vi "Optionen Cluster Anordnen.vi"(8 "error in (no error)":errorcluster caption="Fehler (Eingang, kein Fehler)", 11 "Cluster (Eingang)":refnum<vi>) -> (0 "error out":errorcluster caption="Fehler (Ausgang)", 3 "Numerisch":i32)   [LabVIEW 2020, in "System Einstellungen V2.lvlib"]
uses:
  System Einstellungen V2.lvlib
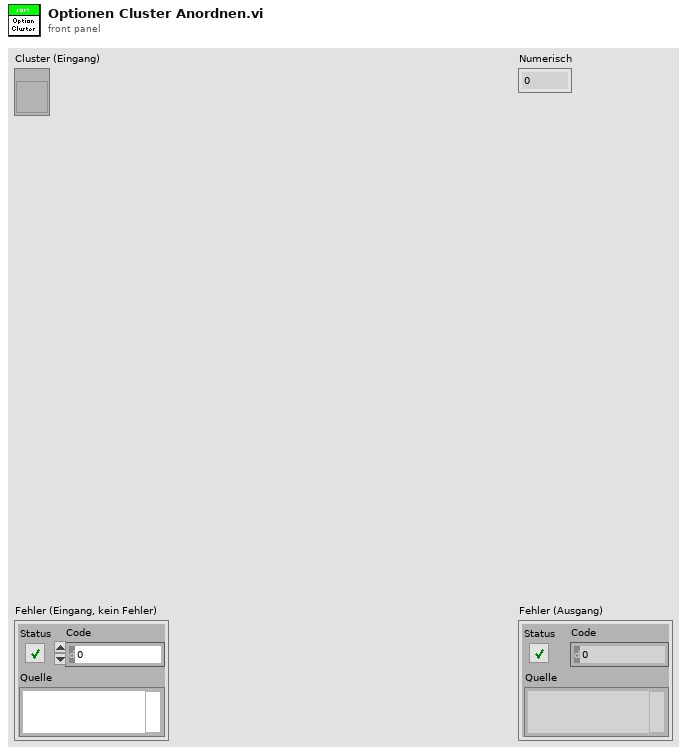
[diagram p1: front panel]
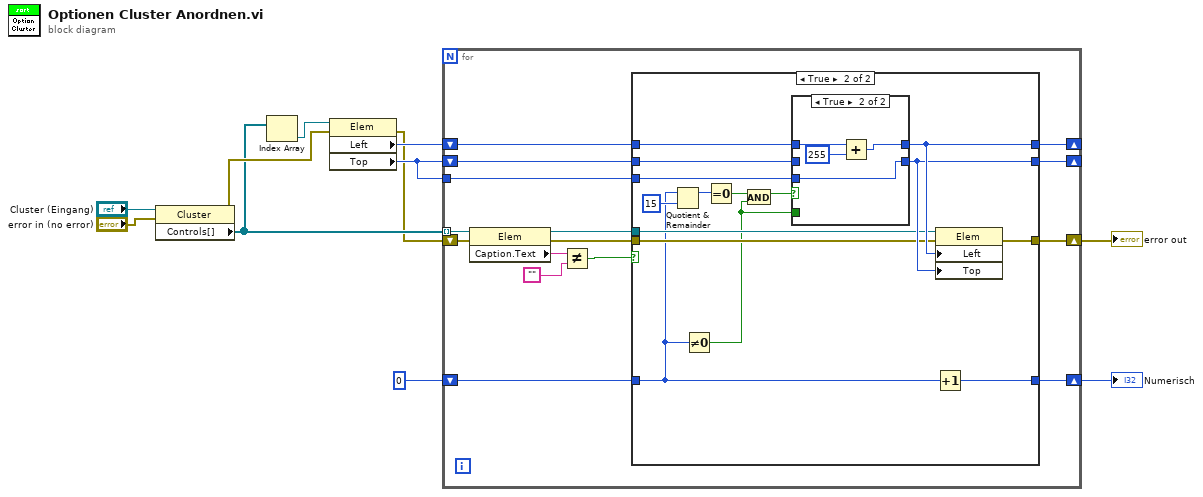
[diagram p0: block diagram]
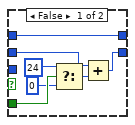
[diagram p3: hidden frame]
diagram:
  n1 = property class="Cluster"(reference="Cluster (Eingang)", error in="error in (no error)") -> (error out=w9:errorcluster, "Controls[]"=w7:refnum<vi>[])  [unwired: 1 out]
  n2 = Index Array(array=w7) -> (element=w10:refnum<vi>)  [unwired: 1 in]
  n3 = property class="Elem"(reference=w10, error in=w9) -> (error out=w3:errorcluster, "Left"=w6:i32, "Top"=w4:i32)  [unwired: 1 out]
  n4 = for {
    tunnel: w7 -> [w18] mode=indexing
    shift-right: [w26] -> w5
    shift-left: w3 -> [w17]
    shift-right: [w23] -> _
    shift-left: w6 -> [w25]
    shift-right: [w22] -> _
    shift-left: w4 -> [w24]
    tunnel: w4 -> [w21]
    shift-right: [w14] -> w1
    shift-left: 0 -> [w16]
    n5 = property class="Elem"(reference=w18, error in=w17) -> (reference out=w12:refnum<vi>, error out=w13:errorcluster, "Caption.Text"=w20:string)
    n6 = Not Equal?(x=w20, y="") -> (x != y?=w15:bool)
    n7 = case shown="True" w15 {
      tunnel: [w29 w45] -> w26
      tunnel: w25 -> [w28 w41]
      tunnel: w24 -> [w27 w40]
      tunnel: [w28 w39] -> w23
      tunnel: [w27 w38] -> w22
      tunnel: w21 -> [_ w37]
      tunnel: w16 -> [w30 w33]
      tunnel: [w30 w36] -> w14
      tunnel: w13 -> [w29 w35]
      tunnel: w12 -> [_ w34]
      frame False {
      }
      frame True {
        n8 = Quotient & Remainder(x=w33, y=15) -> (x-y*floor(x/y)=w43:i32)  [unwired: 1 out]
        n9 = Not Equal To 0?(x=w33) -> (x != 0?=w31:bool)
        n10 = Equal To 0?(x=w43) -> (x = 0?=w42:bool)
        n11 = And(x=w42, y=w31) -> (x .and. y?=w32:bool)
        n12 = case shown="True" w32 {
          tunnel: w41 -> [w52 w55]
          tunnel: w40 -> [w51 _]
          tunnel: [w52 w53] -> w39
          tunnel: [w50 w56] -> w38
          tunnel: w37 -> [_ w56]
          tunnel: w31 -> [w48 _]
          frame False {
            n13 = Select(t=24 ("y"), s=w48, f=0) -> (s? t:f=w49:i32)
            n14 = Add(x=w51, y=w49) -> (x+y=w50:i32)
          }
          frame True {
            n15 = Add(x=w55, y=255) -> (x+y=w53:i32)
          }
        }
        n16 = Increment(x=w33) -> (x+1=w36:i32)
        n17 = property class="Elem"(reference=w34, error in=w35, "Left"=w39, "Top"=w38) -> (error out=w45:errorcluster)  [unwired: 1 out]
      }
    }
  }
  "error out" <- w5
  "Numerisch" <- w1
